vi "linking.vi"() -> ()   [LabVIEW 2016]
panel:
  in  "ActiveX Container":refnum<k7>(container)
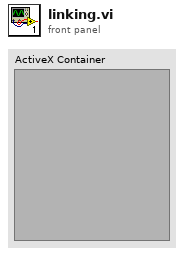
[diagram p1: front panel]
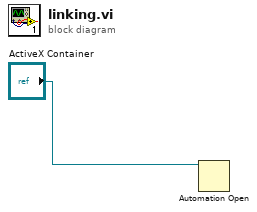
[diagram p0: block diagram]
diagram:
  n1 = Automation Open(Automation Refnum="ActiveX Container") -> ()  [unwired: 3 in, 2 out]
